vi "ASK Transmitter.vi"() -> ()   [LabVIEW 2015]
uses:
  <instrlib>/niUSRP/niUSRP Write Tx Data (CDB).vi
panel:
  out "Transmitted Signal":dbl[](graph)
  in  "Sampling Frequency":dbl
  in  "Data Frequency":dbl
  in  "Iterations":i32
  in  "y":bool
  out "error out":errorcluster
  out "coerced IQ rate":dbl=100000.0 format="%#_6p"
  out "coerced carrier frequency":dbl=100000.0 format="%#_6p"
  out "coerced gain":dbl format="%#_6f"
  in  "IQ rate":dbl=100000.0 format="%#_6p"
  in  "carrier frequency":dbl=100000.0 format="%#_6p"
  in  "gain":dbl format="%#_6f"
  in  "active antenna":string
  in  "device names":refnum<k15>
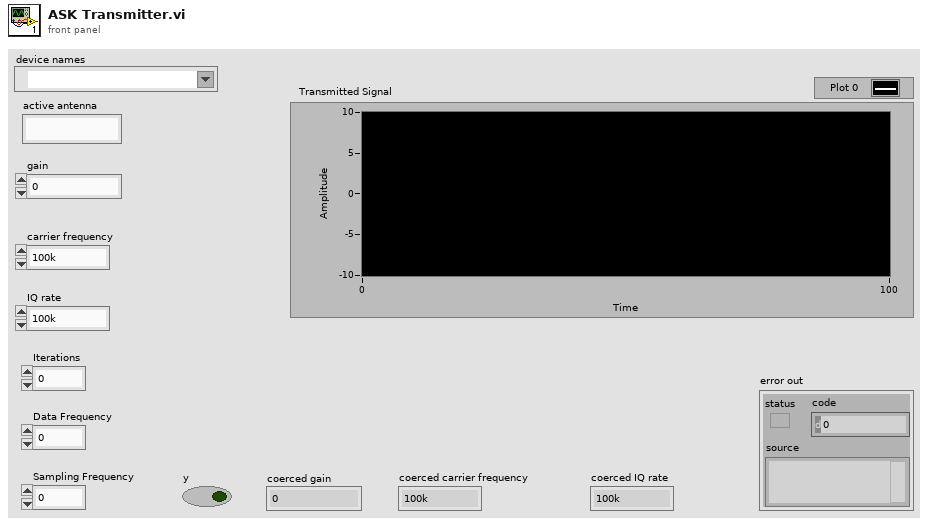
[diagram p1: front panel]
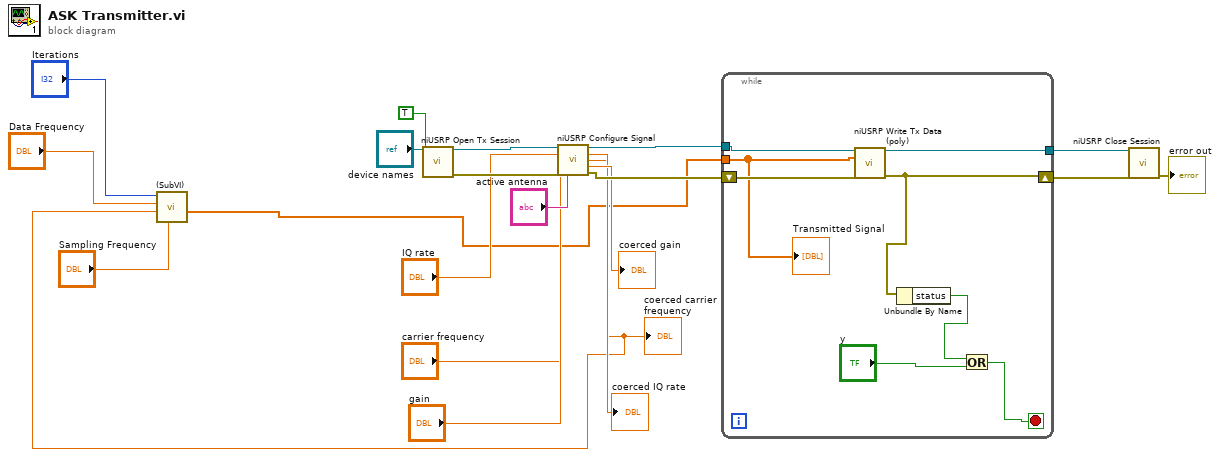
[diagram p0: block diagram]
diagram:
  n1 = call <instrlib>:"niUSRP Open Tx Session.vi"("device names"="device names", "reset"=TRUE) -> ("session handle out"=w19:refnum<k15>, "error out"=w18:errorcluster)  [unwired: 12 in]
  n2 = call <instrlib>:"niUSRP Configure Signal.vi"("session handle"=w19, "IQ rate"="IQ rate", "carrier frequency"="carrier frequency", "gain"="gain", "error in (no error)"=w18, "active antenna"="active antenna") -> ("session handle out"=w9:refnum<k15>, "coerced IQ rate"=→"coerced IQ rate":dbl, "coerced carrier frequency"=w3:dbl, "coerced gain"=→"coerced gain":dbl, "error out"=w12:errorcluster)  [unwired: 5 in]
  "coerced carrier frequency" <- w3
  n3 = call "(SubVI).vi"("Sampling Frequency"="Sampling Frequency", "Carrier Frequency"=w3, "Data Frequency"="Data Frequency", "Iterations"="Iterations") -> ("Modulated Signal"=w1:dbl[])  [unwired: 4 in, 3 out]
  n4 = while {
    shift-right: [w25] -> w8
    shift-left: w12 -> [w28]
    tunnel: w9 -> [w27]
    tunnel: [w26] -> w7
    tunnel: w1 -> [w21]
    stop <- w22 stop-if-true
    n5 = call-poly <instrlib>:"niUSRP Write Tx Data (poly).vi"("session handle"=w27, "data"=w21, "error in (no error)"=w28) -> ("session handle out"=w26:refnum<k15>, "error out"=w25:errorcluster)  [unwired: 11 in]
    n6 = Unbundle By Name(w25) -> ("status"=w24:bool)
    n7 = Or(x=w24, y="y") -> (x .or. y?=w22:bool)
    "Transmitted Signal" <- w21
  }
  n8 = call <instrlib>:"niUSRP Close Session.vi"("session handle"=w7, "error in (no error)"=w8) -> ("error out"=→"error out":errorcluster)  [unwired: 13 in]
